vi "LeakWarningDesktop.vi"(1 "error in (no error)":errorcluster) -> (0 "error out":errorcluster)   [LabVIEW 2013]
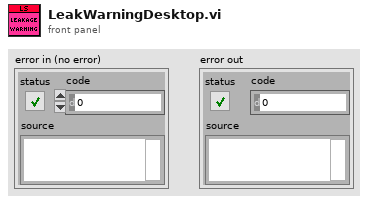
[diagram p1: front panel]
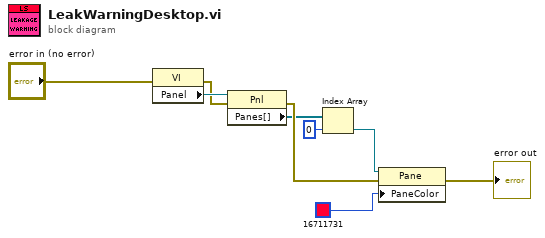
[diagram p0: block diagram]
diagram:
  n1 = property class="VI"(error in="error in (no error)") -> (error out=w6:errorcluster, "Panel"=w7:refnum<vi>)  [unwired: 1 in, 1 out]
  n2 = property class="Pnl"(reference=w7, error in=w6) -> (error out=w5:errorcluster, "Panes[]"=w3:refnum<vi>[])  [unwired: 1 out]
  n3 = Index Array(array=w3, index=0) -> (element=w2:refnum<vi>)
  n4 = property class="Pane"(reference=w2, error in=w5, "PaneColor"=u32 16711731) -> (error out=→"error out":errorcluster)  [unwired: 1 out]
